vi "Assignment #5 Sarah Bailey.vi"() -> ()   [LabVIEW 2013]
panel:
  out "XY Graph":cluster{dbl[], dbl[]}[](graph)
  in  "Table Of Plots":string[][](table)
  # "Developed by: Sarah Bailey\nEngineering Applications Lab\nAssignment #5\nWorked with: \nClair Cunningham\nAlex Offredi\nSteven Smith"
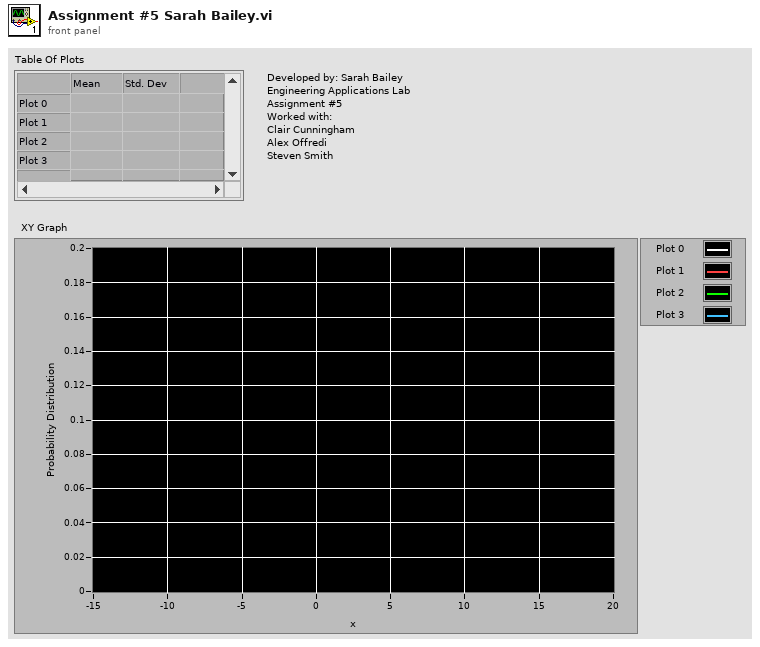
[diagram p1: front panel]
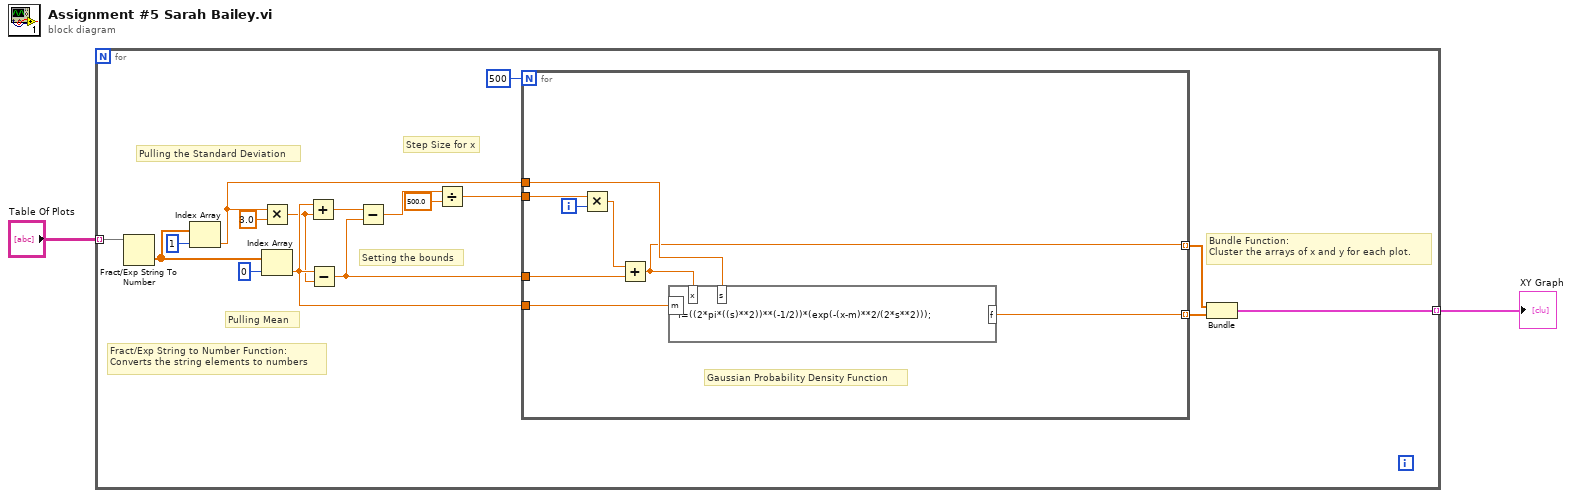
[diagram p0: block diagram]
diagram:
  n1 = for {
    tunnel: "Table Of Plots" -> [w15] mode=indexing
    tunnel: [w8] -> w1 mode=indexing
    # "Setting the bounds"
    # "Bundle Function:\nCluster the arrays of x and y for each plot."
    # "Step Size for x"
    # "Fract/Exp String to Number Function:\nConverts the string elements to numbers"
    # "Pulling the Standard Deviation"
    # "Pulling Mean"
    n2 = Fract/Exp String To Number(string=w15) -> (number=w18:dbl[])  [unwired: 3 in, 1 out]
    n3 = Index Array(array=w18, index=1) -> (element=w4:dbl)
    n4 = Multiply(x=w4, y=3.0) -> (x*y=w3:dbl)
    n5 = Index Array(array=w18, index=0) -> (element=w5:dbl)
    n6 = Add(x=w5, y=w3) -> (x+y=w13:dbl)
    n7 = Subtract(x=w5, y=w3) -> (x-y=w9:dbl)
    n8 = Subtract(x=w13, y=w9) -> (x-y=w12:dbl)
    n9 = Divide(x=w12, y=500.0) -> (x/y=w10:dbl)
    n10 = for {
      N: 500 -> [_]
      tunnel: w5 -> [w27]
      tunnel: w4 -> [w26]
      tunnel: w10 -> [w24]
      tunnel: w9 -> [w25]
      tunnel: [w21] -> w6 mode=indexing
      tunnel: [w20] -> w7 mode=indexing
      i -> [w23]
      # "Gaussian Probability Density Function"
      n11 = Multiply(x=w24, y=w23) -> (x*y=w22:dbl)
      n12 = Add(x=w22, y=w25) -> (x+y=w20:dbl)
      n13 = formula code="f=((2*pi*((s)**2))**(-1/2))*(exp(-(x-m)**2/(2*s**2)));"("s"=w26, "x"=w20, "m"=w27) -> ("f"=w21:dbl)
    }
    n14 = Bundle(w7, w6) -> (w8:cluster{dbl[], dbl[]})  [unwired: 1 in]
  }
  "XY Graph" <- w1
